vi "CheckAndGet_Float2D_data.vi"(0 "data in":sgl[][](array[numeric]), 5 "Dimensions_um":T1) -> (4 "data out":sgl[][](array[numeric]))   [LabVIEW 2020]
uses:
  Controls/General dimensions definition.ctl
  Controls/Point2D.ctl
  Controls/Point2Df.ctl
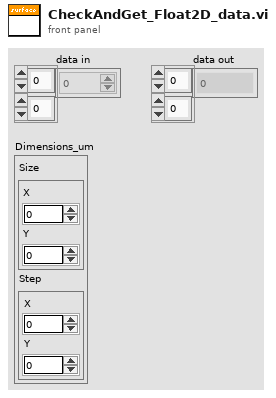
[diagram p1: front panel]
types:
  T1 = typedef "General dimensions definition.ctl" = cluster{"Size":T2, "Step":T3}
  T2 = typedef "Point2D.ctl" = cluster{"X":u32, "Y":u32}
  T3 = typedef "Point2Df.ctl" = cluster{"X":sgl, "Y":sgl}
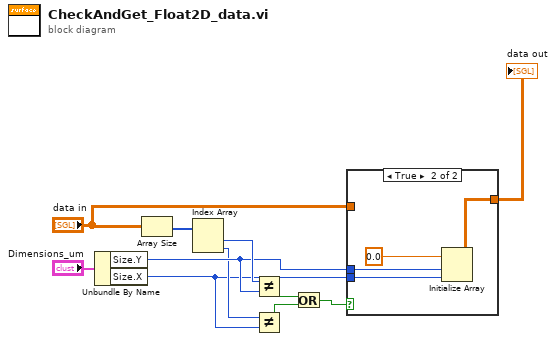
[diagram p0: block diagram]
diagram:
  n1 = Unbundle By Name("Dimensions_um") -> ("Size.Y"=w6:u32, "Size.X"=w4:u32)
  n2 = Array Size(array="data in") -> (size(s)=w8:i32[])
  n3 = Index Array(array=w8) -> (element #1=w7:i32, element #2=w5:i32)  [unwired: 2 in]
  n4 = Not Equal?(x=w7, y=w6) -> (x != y?=w3:bool)
  n5 = Not Equal?(x=w5, y=w4) -> (x != y?=w2:bool)
  n6 = Or(x=w3, y=w2) -> (x .or. y?=w1:bool)
  n7 = case shown="True" w1 {
    tunnel: [w12 w14] -> w10
    tunnel: w6 -> [_ w16]
    tunnel: w4 -> [_ w15]
    tunnel: "data in" -> [w12 _]
    frame False {
    }
    frame True {
      n8 = Initialize Array(sgl 0.0, w16, w15) -> (w14:sgl[][])
    }
  }
  "data out" <- w10
